vi "DAQ_clean_daq.vi"(3 "Error In":errorcluster, 5 "DAQ Settings":T1={"Shutters Settings"=[{"Name"="Shutter 1", "DAQ Channel/line"="Dev1/port0/line0", "Active"=FALSE}, {"Name"="Shutter 2", "DAQ Channel/line"="Dev1/port0/line1", "Active"=FALSE}], "Shutter Task"="", "Acquire Settings"=[], "AI Task"="", "Sample mode"=10178, "Number of Samples"=0, "Rate"=0.0, "AI Name"="", "DO Name"=""} {"Sample mode" items=["Finite Samples"=10178, "Continuous Samples"=10123, "Hardware Timed Single Point"=12522]; "Acquire Settings"."input terminal configuration" items=["default"=-1, "RSE"=10083, "NRSE"=10078, "Differential"=10106, "Pseudodifferential"=12529]}) -> (0 "Error Out":errorcluster)   [LabVIEW 2018]
uses:
  Type defs/DAQ_set_Ctrl.ctl
  Type defs/DAQ_Shutter_Ctrl.ctl
  Type defs/DAQ_AI_Ctrl.ctl
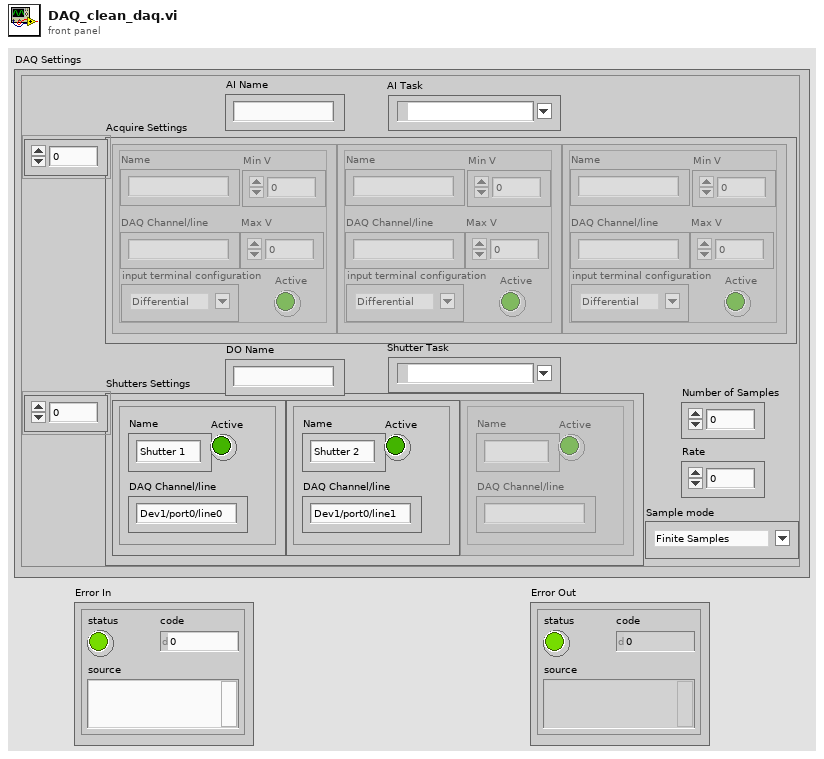
[diagram p1: front panel]
types:
  T1 = typedef "DAQ_set_Ctrl.ctl" = cluster{"Shutters Settings":T2[], "Shutter Task":refnum<k21>, "Acquire Settings":T3[], "AI Task":refnum<k21>, "Sample mode":i32, "Number of Samples":i32, "Rate":dbl, "AI Name":string, "DO Name":string}
  T2 = typedef "DAQ_Shutter_Ctrl.ctl" = cluster{"Name":string, "DAQ Channel/line":string, "Active":bool}
  T3 = typedef "DAQ_AI_Ctrl.ctl" = cluster{"Name":string, "DAQ Channel/line":string, "Max V":dbl, "Min V":dbl, "input terminal configuration":i32, "Active":bool}
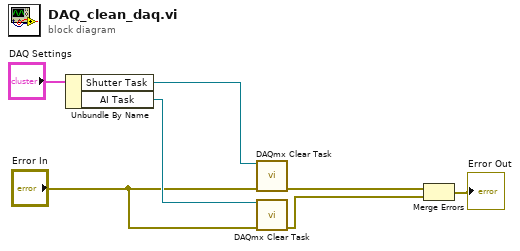
[diagram p0: block diagram]
diagram:
  n1 = Unbundle By Name("DAQ Settings") -> ("Shutter Task"=w6:refnum<k21>, "AI Task"=w5:refnum<k21>)
  n2 = call <vilib>:"DAQmx Clear Task.vi"("task in"=w6, "error in"="Error In") -> ("error out"=w3:errorcluster)  [unwired: 13 in]
  n3 = call <vilib>:"DAQmx Clear Task.vi"("task in"=w5, "error in"="Error In") -> ("error out"=w1:errorcluster)  [unwired: 13 in]
  n4 = Merge Errors(w3, w1) -> (→"Error Out":errorcluster)
